vi "BRig_dataTrial_Cue2_I_High_Sel.vi"() -> (2 "output_Cue2_I_High_Sel":i32)   [LabVIEW 2014]
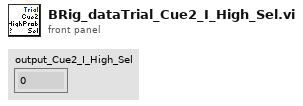
[diagram p1: front panel]
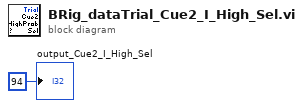
[diagram p0: block diagram]
diagram:
  "output_Cue2_I_High_Sel" <- 94 ("output_iBlock")
